vi "UDP_Stream(FIFO).vi"() -> ()   [LabVIEW 2015]
uses:
  <vilib>/FPGAPlugInAG/cRIO-9063/niLvFpga_Open_cRIO-9063.vi
  <vilib>/rvi/interface/common/dynamic/niFpgaDynamicAddResources.vi
  <vilib>/Utility/error.llb/Error Cluster From Error Code.vi
  <vilib>/rvi/errors/niLvFpgaAdjustHostInterfaceError.vi
  <vilib>/FPGAPlugInAG/Dynamic/niLvFpga_Run_Dynamic.vi
  <vilib>/FPGAPlugInAG/Dynamic/niLvFpga_Close_Dynamic.vi
  <vilib>/rvi/interface/nirviOpenFPGA/nirviOpenFPGA.xnode
  FPGA Bitfiles/VCU-VEHICLEMODEL_FPGATarget_CANBasic(FPGA)_WVt1gIpoBPw.lvbitx
  Basic (FPGA) CAN Engine .vi
  <vilib>/rvi/interface/nirviMethod/nirviMethod.xnode
  <vilib>/rvi/interface/nirviReadWriteControl/nirviReadWriteControl.xnode
  <vilib>/rvi/interface/nirviCloseFPGA/nirviCloseFPGA.xnode
  NiFpgaLv.dll
  <vilib>/rvi/interface/Simulation/niFpgaSimulationCallBeginRW.vi
  <vilib>/FPGAPlugInAG/Dynamic/niLvFpga_ReadFifo_Dynamic.vi
  <vilib>/rvi/errors/niLvFpgaMergeErrorWithErrorCode.vi
  <vilib>/FPGAPlugInAG/Dynamic/niLvFpga_StartFifo_Dynamic.vi
panel:
  out "data string":string
  out "Data":u32[](array[numeric])
  out "Overflow - Timed Out":bool
  in  "Stream":bool
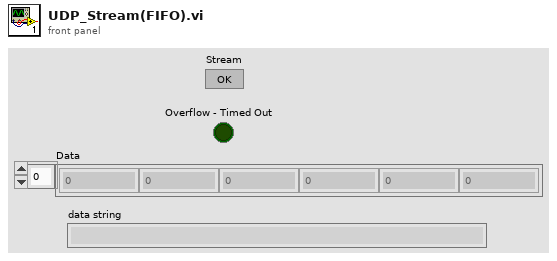
[diagram p1: front panel]
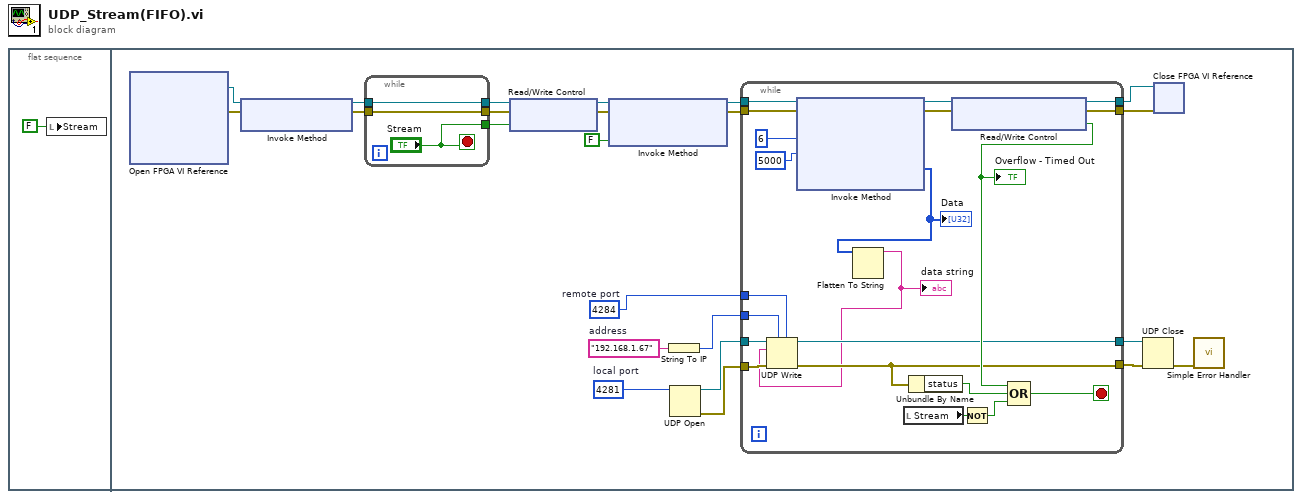
[diagram p0: block diagram]
diagram:
  n1 = flat-sequence {
    frame #0 {
      n2 = local write "Stream"(FALSE ("Stream")) -> ()
    }
    frame #1 {
      w2 = u16 4284  # remote port
      w9 = u16 4281  # local port
      w10 = "192.168.1.67"  # address
      n3 = xnode "Open FPGA VI Reference"() -> ("FPGA VI Reference Out"=w18:refnum<k20>, "error out"=w19:errorcluster)  [unwired: 2 in]
      n4 = xnode "Invoke Method"("FPGA VI Reference In"=w18, "error in"=w19) -> ("FPGA VI Reference Out"=w17:refnum<k20>, "error out"=w16:errorcluster)
      n5 = while {
        tunnel: [w26] -> w24
        tunnel: [w27] -> w23
        tunnel: ["Stream"] -> w20
        tunnel: w17 -> [w27]
        tunnel: w16 -> [w26]
        stop <- "Stream" stop-if-true
      }
      n6 = xnode "Read/Write Control"("FPGA VI Reference In"=w23, "error in"=w24, "Log to buffer"=w20) -> ("FPGA VI Reference Out"=w15:refnum<k20>, "error out"=w13:errorcluster)
      n7 = xnode "Invoke Method"("FPGA VI Reference In"=w15, "error in"=w13, "Wait Until Done (F)"=FALSE) -> ("FPGA VI Reference Out"=w14:refnum<k20>, "error out"=w12:errorcluster)
      n8 = String To IP(1:w10) -> (0:w6:u32)
      n9 = UDP Open(11:w9) -> (port=w7:refnum<k16>, 0:w8:errorcluster)  [unwired: 4 in, 1 out]
      n10 = while {
        tunnel: w14 -> [w48]
        tunnel: w12 -> [w47]
        tunnel: [w34] -> w4
        tunnel: [w43] -> w22
        tunnel: [w41] -> w21
        tunnel: w8 -> [w35]
        tunnel: w7 -> [w33]
        tunnel: [w32] -> w5
        tunnel: w6 -> [w31]
        tunnel: w2 -> [w30]
        stop <- w39 stop-if-true
        n11 = xnode "Invoke Method"("FPGA VI Reference In"=w48, "error in"=w47, "Number of Elements"=u32 6, "Timeout (ms)"=5000) -> ("FPGA VI Reference Out"=w44:refnum<k20>, "error out"=w42:errorcluster, "Data"=w29:u32[])  [unwired: 1 out]
        "Data" <- w29
        n12 = Flatten To String(anything=w29) -> (data string=w28:string)  [unwired: 3 in, 2 out]
        "data string" <- w28
        n13 = UDP Write(address=w31, port or service name=w30, connection ID=w33, data in=w28, 8:w35) -> (error out=w34:errorcluster, 3:w32:refnum<k16>)  [unwired: 1 in]
        n14 = local read "Stream"() -> (w37:bool)
        n15 = Unbundle By Name(w34) -> ("status"=w40:bool)
        n16 = xnode "Read/Write Control"("FPGA VI Reference In"=w44, "error in"=w42) -> ("FPGA VI Reference Out"=w43:refnum<k20>, "error out"=w41:errorcluster, "Overflow - Timed Out"=w38:bool)
        "Overflow - Timed Out" <- w38
        n17 = Not(x=w37) -> (.not. x?=w36:bool)
        n18 = Compound Arithmetic op=OR(w38, w40, w36) -> (w39:bool)
      }
      n19 = UDP Close(connection ID=w5, 8:w4) -> (error out=w3:errorcluster)  [unwired: 1 out]
      n20 = xnode "Close FPGA VI Reference"("FPGA VI Reference In"=w22, "error in"=w21) -> ()  [unwired: 1 out]
      n21 = call <vilib>:"Simple Error Handler.vi"("error in (no error)"=w3) -> ()  [unwired: 4 in, 5 out]
    }
  }
